vi "Get ClassName, PropNames and Versions.vi"(10 "object":refnum<class "_ISerializable.lvclass">) -> (1 "versions":string[](array[string]), 2 "Class Names":string[](array[string]))   [LabVIEW 2018, in "ORM Scripter.lvclass"]
uses:
  ORM Scripter.lvclass
  _Serializable Base Object/_ISerializable.lvclass
  demo/Implementations/Product-A.lvclass
panel:
  out "names":string[][](array[string])
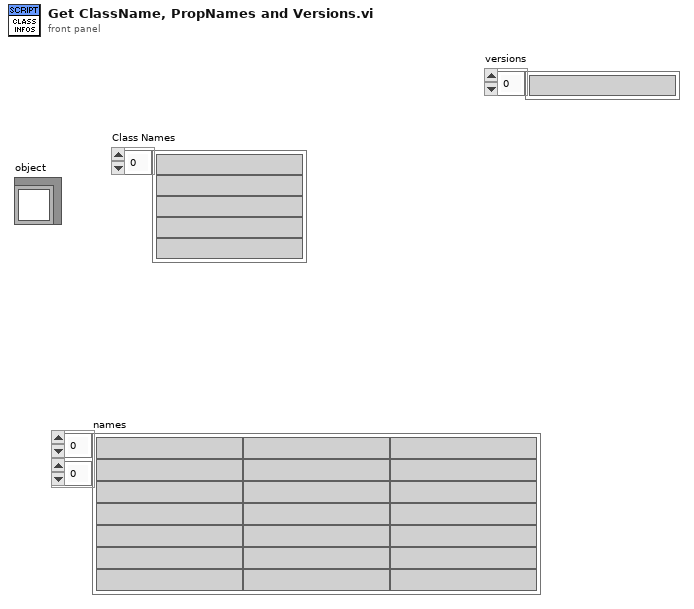
[diagram p1: front panel]
types:
  T1 = cluster{"Major":u16, "Minor":u16, "Fix":u16, "Build":u16}
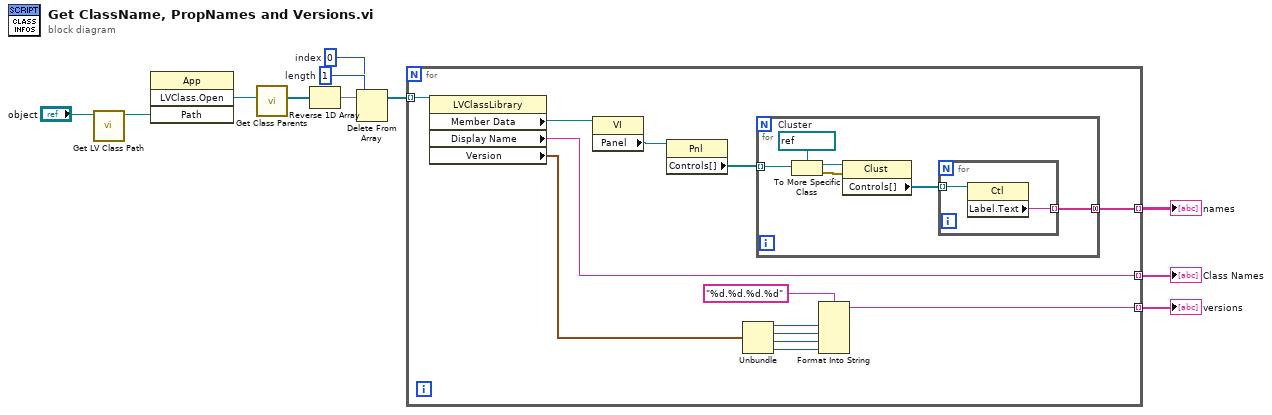
[diagram p0: block diagram]
diagram:
  w3 = 0  # index
  w4 = 1  # length
  n1 = call <vilib>:"Get LV Class Path.vi"("object"="object") -> ("class path"=w11:path)  [unwired: 9 in, 1 out]
  n2 = invoke class="App" method="LVClass.Open"("Path"=w11) -> ("LVClass.Open"=w9:refnum<vi>)  [unwired: 3 in, 3 out]
  n3 = call "Get Class Parents.vi"("LVClassLibrary in"=w9) -> ("Array"=w8:refnum<vi>[])  [unwired: 9 in, 1 out]
  n4 = Reverse 1D Array(array=w8) -> (reversed array=w6:refnum<vi>[])
  n5 = Delete From Array(array=w6, length=w4, index=w3) -> (array with subset deleted=w5:refnum<vi>[])  [unwired: 1 out]
  n6 = for {
    tunnel: w5 -> [w21] mode=indexing
    tunnel: [w20] -> w10 mode=indexing
    tunnel: [w19] -> w2 mode=indexing
    tunnel: [w12] -> w7 mode=indexing
    n7 = property class="LVClassLibrary"(reference=w21) -> ("Member Data"=w23:refnum<vi>, "Display Name"=w19:string, "Version"=w18:T1)  [unwired: 1 in, 2 out]
    n8 = property class="VI"(reference=w23) -> ("Panel"=w24:refnum<vi>)  [unwired: 1 in, 2 out]
    n9 = property class="Pnl"(reference=w24) -> ("Controls[]"=w22:refnum<vi>[])  [unwired: 1 in, 2 out]
    n10 = Unbundle(w18) -> ("Major"=w17:u16, "Minor"=w14:u16, "Fix"=w15:u16, "Build"=w16:u16)
    n11 = for {
      tunnel: w22 -> [w25] mode=indexing
      tunnel: [w27] -> w20 mode=concatenating
      w30 = refnum<vi> refnum  # Cluster
      n12 = To More Specific Class(target class=w30, reference=w25) -> (specific class reference=w29:refnum<vi>, error out=w28:errorcluster)  [unwired: 1 in]
      n13 = property class="Clust"(reference=w29, error in=w28) -> ("Controls[]"=w26:refnum<vi>[])  [unwired: 2 out]
      n14 = for {
        tunnel: w26 -> [w32] mode=indexing
        tunnel: [w31] -> w27 mode=indexing
        n15 = property class="Ctl"(reference=w32) -> ("Label.Text"=w31:string)  [unwired: 1 in, 2 out]
      }
    }
    n16 = Format Into String(format string="%d.%d.%d.%d", w17, w14, w15, w16) -> (resulting string=w12:string)  [unwired: 2 in, 1 out]
  }
  "names" <- w10
  "Class Names" <- w2
  "versions" <- w7
